vi "Test Parse.vi"() -> ()   [LabVIEW 2020]
uses:
  NMEA/NMEA_Type.ctl
  GPS/GPS.lvclass
  C:/Users/dzoni/Documents/NJ/Playground/LV/TCP GPS/lv_tcp_gps/TCP/TCP.lvclass
  TCP/TCP.lvclass/TCP.ctl
  4bec4c2f-f971-4ce2-8ee6-93cbad333557.vi
  TCP/TCP.lvclass
  NMEA/NMEA.lvlib
panel:
  out "Msg Data":variant[](array[variant])
  out "Msg Types":T1[](array[typedef])
  in  "Stop":bool
  out "ID":string
  out "Port":u16
  out "Data":string
  out "Address":string
  out "error out":errorcluster
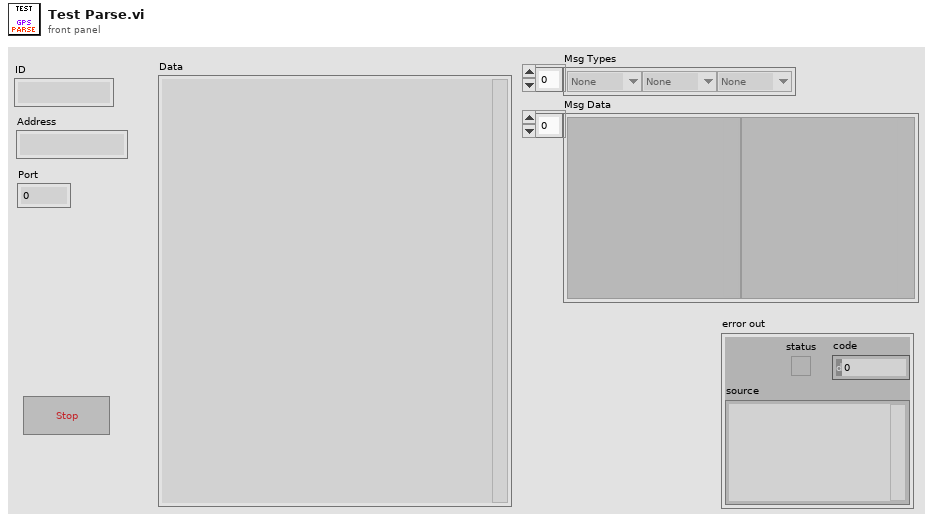
[diagram p1: front panel]
types:
  T1 = typedef "NMEA.lvlib/NMEA_Type.ctl" = enum16{"None", "GGA", "VTG", "RMC"}
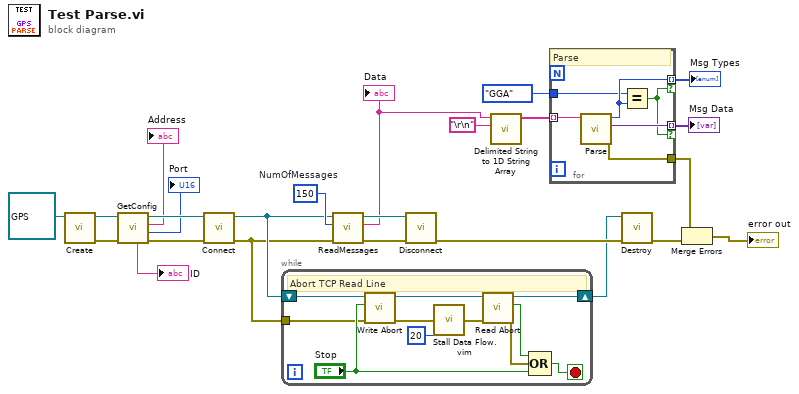
[diagram p0: block diagram]
diagram:
  w13 = 150  # NumOfMessages
  n1 = call-dynamic "Create.vi"("GPS in"=refnum<class "GPS.lvclass"> refnum ("ClientApp1 in")) -> ("error out"=w19:errorcluster, "GPS out"=w21:refnum<class "GPS.lvclass">)  [unwired: 9 in]
  n2 = call "GetConfig.vi"("error in (no error)"=w19, "ClientBase in"=w21) -> ("error out"=w18:errorcluster, "Port"=→"Port":u16, "Address"=→"Address":string, "ClientBase out"=w20:refnum<class "GPS.lvclass">, "ID"=→"ID":string)  [unwired: 5 in]
  n3 = call "Connect.vi"("error in (no error)"=w18, "ClientBase in"=w20) -> ("error out"=w11:errorcluster, "ClientBase out"=w12:refnum<class "GPS.lvclass">)  [unwired: 8 in]
  n4 = while {
    tunnel: w11 -> [w30]
    shift-right: [w26] -> w1
    shift-left: w12 -> [w35]
    stop <- w32 stop-if-true
    # "Abort TCP Read Line"
    n5 = call "Write Abort.vi"("error in (no error)"=w30, "Abort"="Stop", "ClientBase in"=w35) -> ("error out"=w28:errorcluster, "ClientBase out"=w33:refnum<class "GPS.lvclass">)  [unwired: 7 in]
    n6 = call "Stall Data Flow.vim"("value in"=w28, "milliseconds to wait"=u32 20) -> ("value out"=w27:errorcluster)  [unwired: 1 out]
    n7 = call "Read Abort.vi"("error in (no error)"=w27, "ClientBase in"=w33) -> ("error out"=w25:errorcluster, "Abort"=w31:bool, "ClientBase out"=w26:refnum<class "GPS.lvclass">)  [unwired: 7 in]
    n8 = Compound Arithmetic op=OR(w31, w25, "Stop") -> (w32:bool)
  }
  n9 = call "ReadMessages.vi"("error in (no error)"=w11, "NumOfMessages"=w13, "GPS in"=w12) -> ("error out"=w23:errorcluster, "Data"=w7:string, "GPS out"=w24:refnum<class "GPS.lvclass">)  [unwired: 6 in]
  "Data" <- w7
  n10 = call-dynamic "Disconnect.vi"("error in (no error)"=w23, "ClientBase in"=w24) -> ("error out"=w22:errorcluster)  [unwired: 8 in, 1 out]
  n11 = call <vilib>:"Delimited String to 1D String Array.vi"("delimiter"="\r\n", "delimited string"=w7) -> ("string array"=w5:string[])  [unwired: 9 in]
  n12 = for {
    tunnel: [w41] -> w10
    tunnel: w5 -> [w40] mode=indexing
    tunnel: [w39] -> w4 mode=indexing if=w36
    tunnel: NMEA_Type."GGA" ("y") -> [w38]
    tunnel: [w37] -> w2 mode=indexing if=w36
    # "Parse"
    n13 = call "Parse.vi"("MessageStr"=w40) -> ("error out"=w41:errorcluster, "MessageVar"=w37:variant, "MessageType"=w39:T1)  [unwired: 8 in]
    n14 = Equal?(x=w38, y=w39) -> (x = y?=w36:bool)
  }
  "Msg Types" <- w4
  "Msg Data" <- w2
  n15 = call-dynamic "Destroy.vi"("error in (no error)"=w22, "ClientBase in"=w1) -> ("error out"=w8:errorcluster)  [unwired: 9 in]
  n16 = Merge Errors(w10, w8) -> (→"error out":errorcluster)
